vi "Visualise STL file and Octree.vi"() -> ()   [LabVIEW 2015]
doc: "Interactive tool to inspect an STL file and build the Octree for the STL file and check the resulting output. The Octree resolution may be interactively adjusted or set to automatic. The number of branch levels and nodes depends on the geometry, however a rough guide would be to aim for between 5 and 7 branch levels and order 10k nodes."
uses:
  <vilib>/Utility/miscctls.llb/LV3DPointTypeDef.ctl
  <vilib>/Utility/miscctls.llb/LVRGBAColorTypeDef.ctl
  Typedefs/TreeNodeBox.ctl
  Typedefs/Quad.ctl
  Typedefs/Quadplane enum.ctl
  Subroutines/Dot product.vi
panel:
  out "error out":errorcluster
  in  "Camera Controller:Type":T1(ring)=enum."Oriented"
  in  "Autocalc Octree resolution":bool=TRUE
  out "Branch levels":i32
  in  "Scale to unit sphere (render only)":bool
  in  "Octree file path":path=path "C:/EnFlo Software/Anemometry/Anemometry Sub Vis/Collision_Detection/Triangles/Example files/DIPLOS array.oct"
  in  "Render mode":u16(ring)=3 items=["Inherit Value", "Points", "Wireframe", "Polygons"]
  in  "Build Octree":bool
  in  "Draw populated leaf nodes only":bool=TRUE
  out "Number of triangles":u32
  in  "STL file path":path=path "C:/EnFlo Software/Anemometry/Anemometry Sub Vis/Collision_Detection/Triangles/Example files/DIPLOS array.stl"
  in  "Render window":bool=TRUE
  out "Number of Octree nodes":i32
  in  "Octree resolution (model units)":sgl=100.0
  out "Pmin (x, y, z)":sgl[](array[numeric])
  out "Pmax (x, y, z)":sgl[](array[numeric])
  in  "Up Direction":T2={"X"=0.0, "Y"=0.0, "Z"=1.0}
  in  "Target":T2
  in  "Camera Position":T2={"X"=3000.0, "Y"=0.0, "Z"=1000.0}
  out "3D Picture":refnum<vi>(3d-picture)
  # "To view model alone, uncheck \"Build Octree\" and empty \"Octree binary path\".\nTo load Octree after build, uncheck \"Build Octree\"."
  # "PN 03/02/2015"
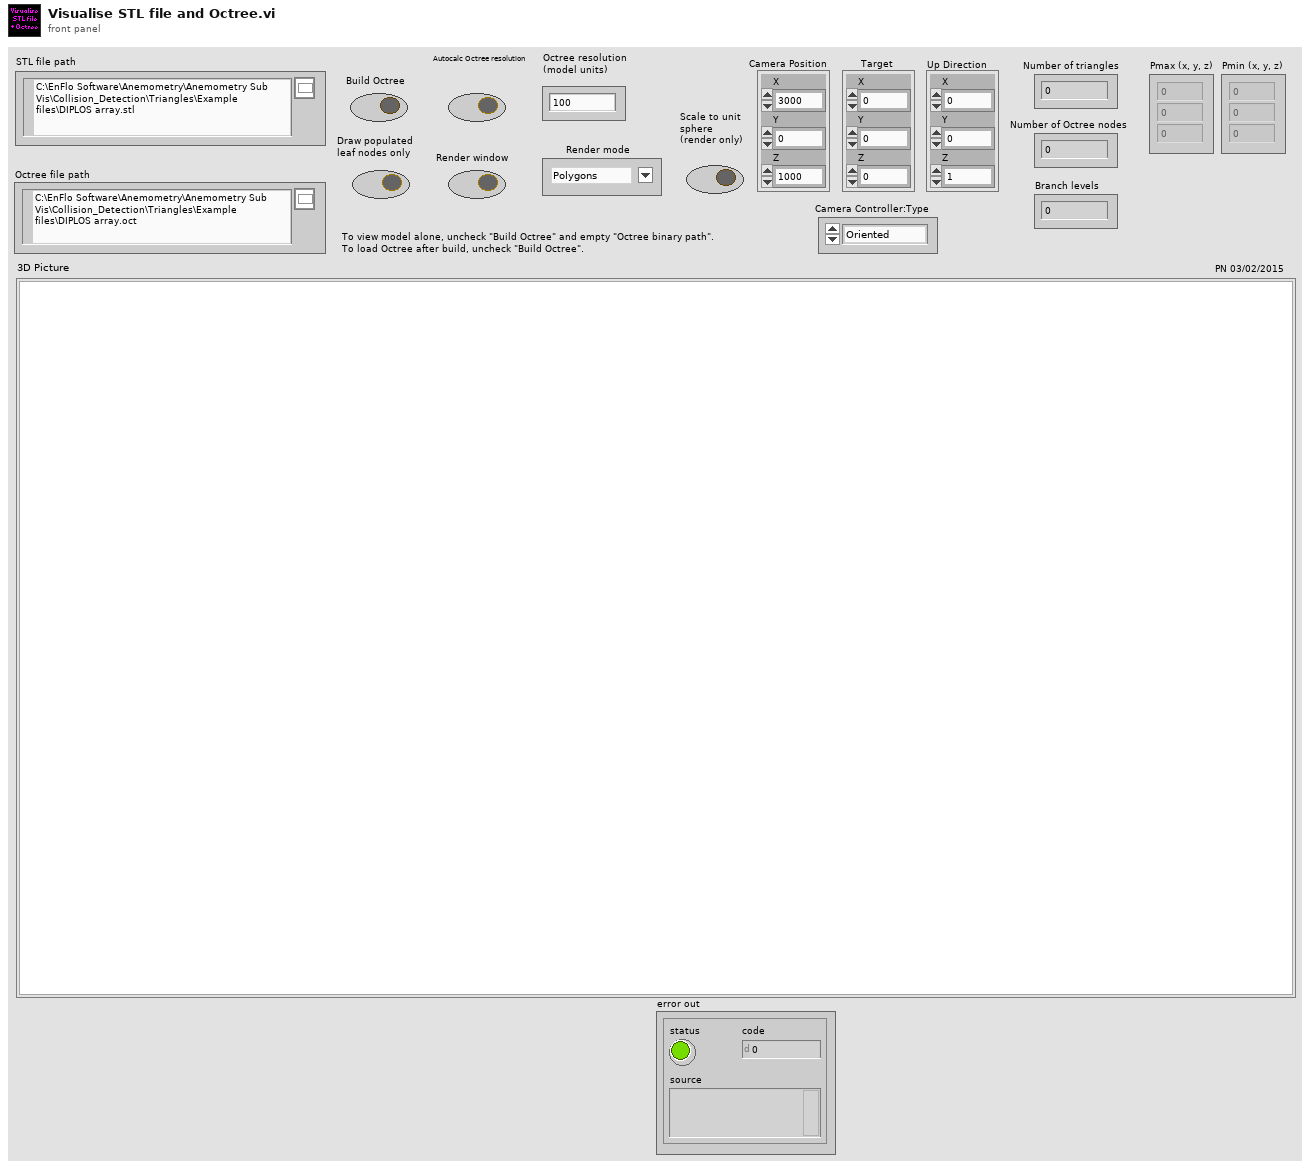
[diagram p1: front panel]
types:
  T1 = enum16{"None", "Spherical", "Flying", "Oriented"}
  T2 = typedef "LV3DPointTypeDef.ctl" = cluster{"X":sgl, "Y":sgl, "Z":sgl}
  T3 = typedef "LVRGBAColorTypeDef.ctl" = cluster{"Red":sgl, "Green":sgl, "Blue":sgl, "Alpha":sgl}
  T4 = typedef "Triangle.ctl" = cluster{"V0":sgl[], "V1":sgl[], "V2":sgl[], "E0":sgl[], "E1":sgl[], "E2":sgl[], "n^":sgl[], "nE0^":sgl[], "nE1^":sgl[], "nE2^":sgl[]}
  T5 = typedef "TreeNodeBox.ctl" = cluster{"Face 0":T6, "Face 1":T6, "Face 2":T6, "Face 3":T6, "Face 4":T6, "Face 5":T6, "Level":i32, "Pmax":sgl[], "Pmin":sgl[], "Parent":i32, "Child 1":i32, "Child 2":i32, "Child 3":i32, "Child 4":i32, "Child 5":i32, "Child 6":i32, "Child 7":i32, "Child 8":i32, "Triangles":i32[], "is leaf node":bool}
  T6 = typedef "Quad.ctl" = cluster{"V0":sgl[], "V1":sgl[], "V2":sgl[], "V3":sgl[], "E0":sgl[], "E1":sgl[], "E2":sgl[], "E3":sgl[], "n^":sgl[], "Plane":T7}
  T7 = typedef "Quadplane enum.ctl" = enum8{"XY", "XZ", "YZ", "-XY", "-XZ", "-YZ"}
  T8 = typedef "LVRectTypeDef.ctl" = cluster{"Left":i16, "Top":i16, "Right":i16, "Bottom":i16}
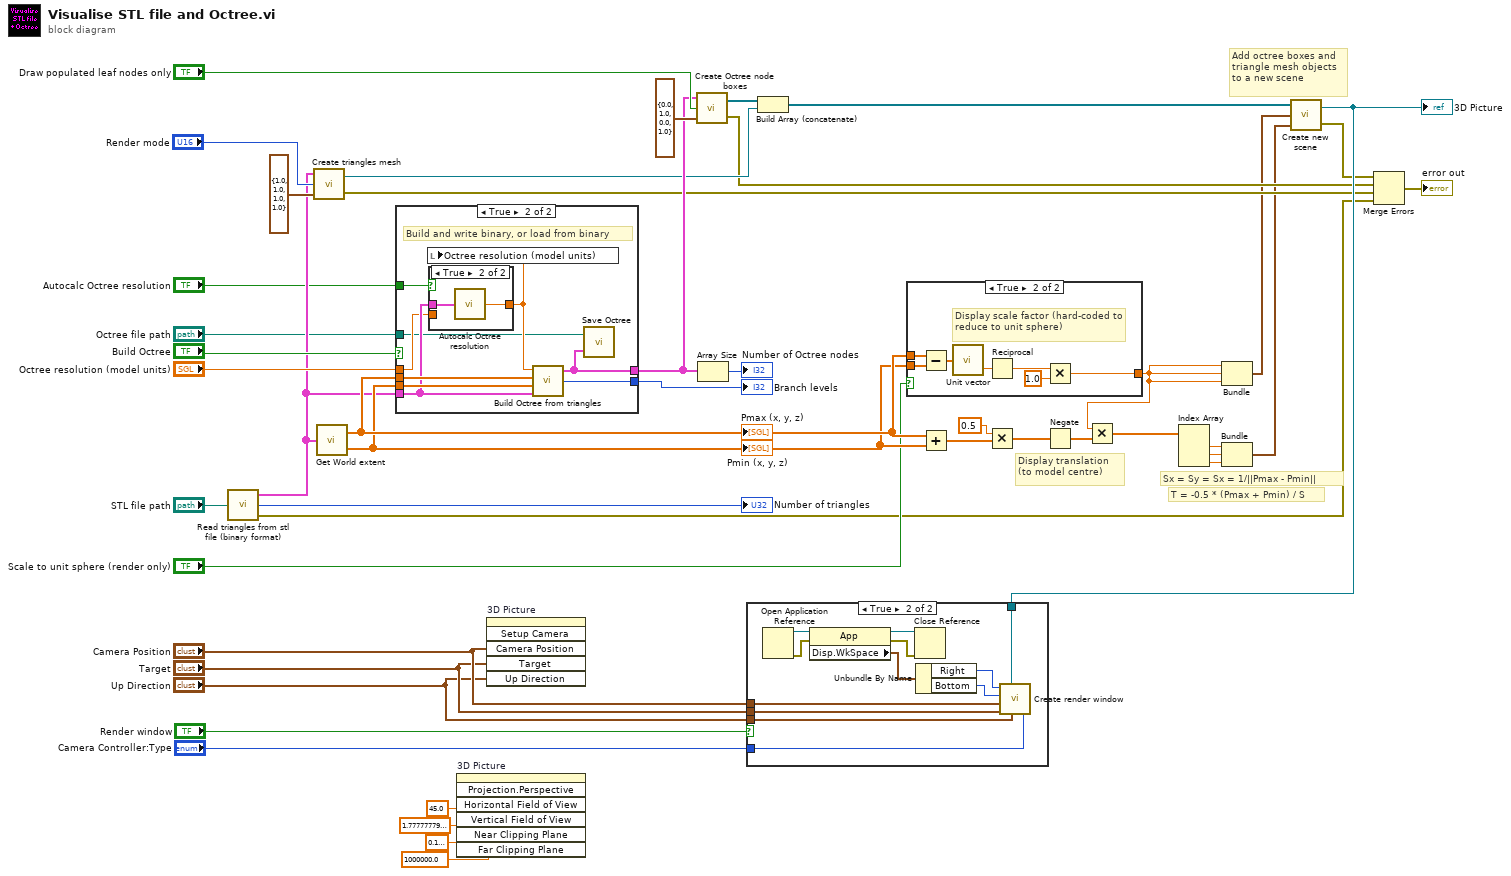
[diagram p0: block diagram]
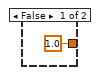
[diagram p3: hidden frame]
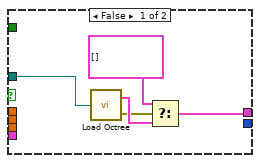
[diagram p4: hidden frame]
diagram:
  # "Add octree boxes and triangle mesh objects to a new scene"
  # "Display translation (to model centre)"
  # "T = -0.5 * (Pmax + Pmin) / S"
  # "Sx = Sy = Sx = 1/||Pmax - Pmin||"
  n1 = call "Read triangles from stl file (binary format).vi"("STL file path"="STL file path") -> ("Triangles array"=w26:T4[], "N triangles"=→"Number of triangles":u32, "Error out"=w4:errorcluster)
  n2 = call "Create triangles mesh.vi"("Colour"=T3 {"Red"=1.0, "Green"=1.0, "Blue"=1.0, "Alpha"=1.0} ("Color"), "Render mode"="Render mode", "Triangles array"=w26) -> ("Error out"=w5:errorcluster, "Triangle mesh out"=w10:refnum<vi>)
  n3 = call "Get World extent.vi"("Triangles"=w26) -> ("Pmax (x, y, z)"=w39:sgl[], "Pmin (x, y, z)"=w38:sgl[])
  "Pmax (x, y, z)" <- w39
  "Pmin (x, y, z)" <- w38
  n4 = case shown="True" "Build Octree" {
    tunnel: "Octree resolution (model units)" -> [_ w54]
    tunnel: w39 -> [_ w60]
    tunnel: w38 -> [_ w59]
    tunnel: [w51 w52] -> w25
    tunnel: w26 -> [_ w56]
    tunnel: "Octree file path" -> [w49 w53]
    tunnel: [_ w58] -> w18
    tunnel: "Autocalc Octree resolution" -> [_ w57]
    frame False {
      n5 = call "Load Octree.vi"("Octree file path"=w49) -> ("Octree node array"=w48:T5[], "Error out"=w47:errorcluster)
      n6 = Select(t=T5[] [], s=w47, f=w48) -> (s? t:f=w51:T5[])
    }
    frame True {
      # "Build and write binary, or load from binary"
      n7 = case shown="True" w57 {
        tunnel: w56 -> [_ w63]
        tunnel: [w61 w62] -> w55
        tunnel: w54 -> [w61 _]
        frame False {
        }
        frame True {
          n8 = call "Autocalc Octree resolution.vi"("Triangles array"=w63) -> ("Suggested resolution"=w62:sgl)
        }
      }
      n9 = local write "Octree resolution (model units)"(w55) -> ()
      n10 = call "Build Octree from triangles.vi"("Triangle array"=w56, "World Pmin (x, y, z)"=w59, "World Pmax (x, y, z)"=w60, "Octree resolution (model units)"=w55) -> ("Branch levels"=w58:i32, "Octree node array"=w52:T5[])  [unwired: 1 out]
      n11 = call "Save Octree.vi"("Octree node array"=w52, "Octree file path"=w53) -> ()  [unwired: 1 out]
    }
  }
  "Branch levels" <- w18
  n12 = invoke on="3D Picture" class="SceneGraphDisp (strict)" method="Projection.Perspective"("Horizontal Field of View"=sgl 45.0 ("Field of View"), "Vertical Field of View"=sgl 1.7777778 ("Aspect Ratio"), "Near Clipping Plane"=sgl 0.1, "Far Clipping Plane"=sgl 1000000.0) -> ()  [unwired: 3 in, 7 out]
  n13 = invoke on="3D Picture" class="SceneGraphDisp (strict)" method="Setup Camera"("Camera Position"="Camera Position", "Target"="Target", "Up Direction"="Up Direction") -> ()  [unwired: 3 in, 6 out]
  n14 = call "Create Octree node boxes.vi"("Colour (emission)"=T3 {"Red"=0.0, "Green"=1.0, "Blue"=0.0, "Alpha"=1.0}, "Draw populated leaf nodes only"="Draw populated leaf nodes only", "Octree nodes array"=w25) -> ("Error out"=w6:errorcluster, "Octree node boxes array"=w11:refnum<vi>[])
  n15 = Array Size(array=w25) -> (size(s)=→"Number of Octree nodes":i32)
  n16 = Build Array (concatenate)(w11, w10) -> (w9:refnum<vi>[])
  n17 = case shown="True" "Scale to unit sphere (render only)" {
    tunnel: w39 -> [_ w71]
    tunnel: w38 -> [_ w70]
    tunnel: [sgl 1.0 w67] -> w35
    frame False {
    }
    frame True {
      # "Display scale factor (hard-coded to reduce to unit sphere)"
      n18 = Subtract(x=w71, y=w70) -> (x-y=w69:sgl[])
      n19 = call "Unit vector.vi"("Vector"=w69) -> ("Vector magnitude"=w66:sgl)  [unwired: 1 out]
      n20 = Reciprocal(x=w66) -> (1/x=w68:sgl)
      n21 = Multiply(x=w68, y=sgl 1.0) -> (x*y=w67:sgl)
    }
  }
  n22 = Add(x=w39, y=w38) -> (x+y=w40:sgl[])
  n23 = Multiply(x=sgl 0.5 ("Numeric"), y=w40) -> (x*y=w34:sgl[])
  n24 = Negate(x=w34) -> (-x=w37:sgl[])
  n25 = Multiply(x=w35, y=w37) -> (x*y=w36:sgl[])
  n26 = Index Array(array=w36) -> (element #1=w44:sgl, element #2=w43:sgl, element #3=w42:sgl)  [unwired: 3 in]
  n27 = Bundle(w35, w35, w35) -> (w2:cluster{sgl, sgl, sgl})  [unwired: 1 in]
  n28 = Bundle(w44, w43, w42) -> (w1:cluster{sgl, sgl, sgl})  [unwired: 1 in]
  n29 = call "Create new scene.vi"("Translation"=w1, "Scale"=w2, "Scene objects array"=w9) -> ("Error out"=w7:errorcluster, "Scene out"=w8:refnum<vi>)
  "3D Picture" <- w8
  n30 = case shown="True" "Render window" {
    tunnel: "Camera Position" -> [_ w83]
    tunnel: "Target" -> [_ w82]
    tunnel: "Up Direction" -> [_ w81]
    tunnel: w8 -> [_ w80]
    tunnel: "Camera Controller:Type" -> [_ w72]
    frame False {
    }
    frame True {
      n31 = Open Application Reference() -> (0:w76:errorcluster, 3:w75:refnum<vi>)  [unwired: 4 in]
      n32 = property class="App"(reference=w75, error in=w76) -> (reference out=w77:refnum<vi>, error out=w78:errorcluster, "Disp.WkSpace"=w79:T8)
      n33 = Close Reference(reference=w77, error in (no error)=w78) -> ()  [unwired: 1 out]
      n34 = Unbundle By Name(w79) -> ("Right"=w73:i16, "Bottom"=w74:i16)
      n35 = call "Create render window.vi"("Camera Controller:Type"=w72, "Up Direction"=w81, "Scene"=w80, "Target"=w82, "Camera Position"=w83, "Height"=w74, "Width"=w73) -> ()  [unwired: 1 in]
    }
  }
  n36 = Merge Errors(w7, w6, w5, w4) -> (→"error out":errorcluster)
